vi "Subscribe.vi"(5 "Message Transport Interface":refnum<class "Message Transport Interface.lvclass">, 6 "Subscriber Name":string, 7 "Topic Name":string, 8 "error in (no error)":errorcluster, 11 "Message Broker Interface TAP in":refnum<class "Message Broker Interface Ref.lvclass">) -> (0 "error out":errorcluster, 2 "Topic Actor Created?":bool, 3 "Message Broker Interface TAP out":refnum<class "Message Broker Interface Ref.lvclass">)   [LabVIEW 2016, in "Stream Mediator.lvlib" / "Message Broker Interface Ref.lvclass"]
doc: "--\nCopyright © 2017 Composed SystemsI All rights reserved.\n\nAuthor: Jon McBee <jon.mcbee@composed.io>\n\nThis library is provided \"AS IS\" ,WITHOUT WARRANTIES OR\nCONDITIONS OF ANY KIND, either express or implied.\n\nComposed Systems -- composed.io\n\nStream 0.0.1.1\nJon McBee - Composed Systems\nCopyright (c) 2017, Composed Systems"
uses:
  <userlib>/Composed Systems/Stream/Mediator/Classes/Message Broker Interface Ref/Message Broker Interface Ref.lvclass
  <userlib>/Composed Systems/Stream/Mediator/Classes/Message Transport Interface/Message Transport Interface.lvclass
  <userlib>/Composed Systems/Stream/Mediator/Classes/Message Broker Interface Ref/Message Broker Interface Ref.lvclass/Message Broker Interface Ref.ctl
  <userlib>/Composed Systems/Stream/Mediator/Classes/Message Broker/Message Broker.lvclass
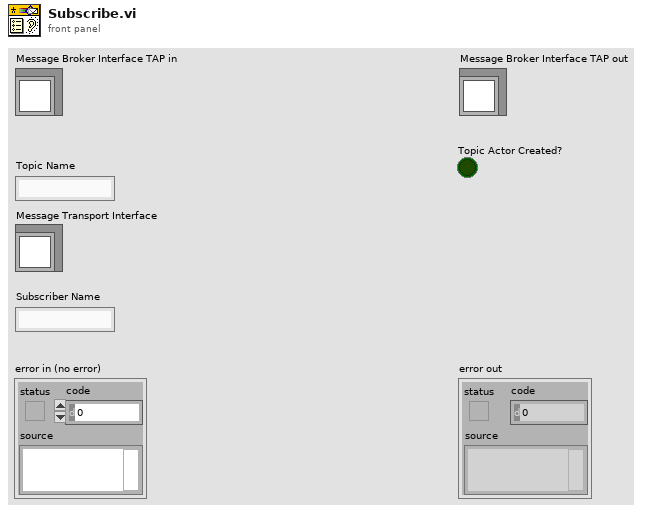
[diagram p1: front panel]
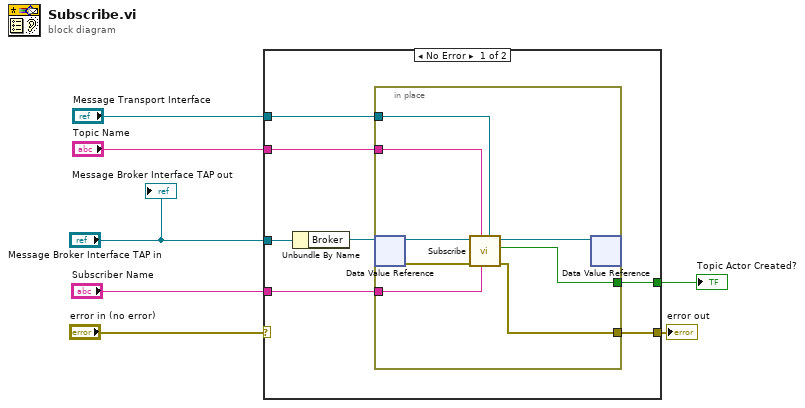
[diagram p0: block diagram]
diagram:
  n1 = case shown="No Error" "error in (no error)" {
    selector: "error in (no error)" -> [_ w23]
    tunnel: "Message Broker Interface TAP in" -> [w14 _]
    tunnel: [w12 w23] -> w5
    tunnel: "Topic Name" -> [w11 _]
    tunnel: "Message Transport Interface" -> [w10 _]
    tunnel: "Subscriber Name" -> [w9 _]
    tunnel: [w8 _] -> w1
    frame No Error {
      n2 = Unbundle By Name(w14) -> ("Broker"=w13:refnum<data-value>)
      n3 = in-place {
        in-place-border: [w19] -> w12
        in-place-border: w11 -> [w18]
        in-place-border: w10 -> [w17]
        in-place-border: w9 -> [w16]
        in-place-border: [w15] -> w8
        n4 = in-place-dvr #1(w13) -> (w22:refnum<class "Message Broker.lvclass">, w20:errorcluster)
        n5 = call <userlib>:"Subscribe.vi"("Message Transport Interface"=w17, "Subscriber Name"=w16, "Topic Name"=w18, "error in (no error)"=w20, "Message Broker in"=w22) -> ("error out"=w19:errorcluster, "Topic Actor Created?"=w15:bool, "Message Broker out"=w21:refnum<class "Message Broker.lvclass">)  [unwired: 4 in]
        n6 = in-place-dvr #1(w21) -> ()  [unwired: 2 out]
      }
    }
    frame Error {
    }
  }
  "error out" <- w5
  "Topic Actor Created?" <- w1
  "Message Broker Interface TAP out" <- "Message Broker Interface TAP in"
